vi "MB Director.vi"(4 "Timeout":u32=1000, 6 "MB Director":T1, 8 "error in (no error)":errorcluster, 11 "MB Port in":refnum<visa-resource-name>) -> (0 "error out":errorcluster, 3 "MB Port out":refnum<visa-resource-name>)   [LabVIEW 2019]
uses:
  MB Director.ctl
  MB cmd buffer.ctl
  MB Serial Master Query Write Multiple Registers (poly).vi
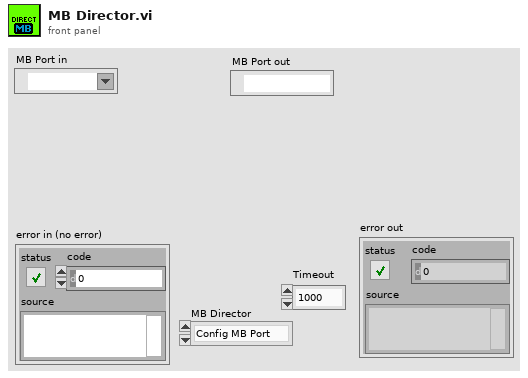
[diagram p1: front panel]
types:
  T1 = typedef "MB Director.ctl" = enum16{"Config MB Port", "Run MB", "Get MB Port", "Quit MB"}
  T2 = typedef "MB cmd buffer.ctl" = enum16{"ProCoDA", "MB", "MB Next Task", "ProCoDA read 1"}
  T3 = typedef "MB ID-Address.ctl" = cluster{"Device ID":u8, "Register":u16}
  T4 = typedef "MB status.ctl" = cluster{"ProCoDA Request":T5, "MB response":dbl[], "new cmd":bool, "error":errorcluster, "MB update(s)":dbl}
  T5 = typedef "ProCoDA MB Request.ctl" = cluster{"# registers":u8, "Data to write":u16[], "data interval (s)":dbl, "command":T6, "PC update (s)":dbl}
  T6 = typedef "Read Write.ctl" = enum16{"Read", "Write"}
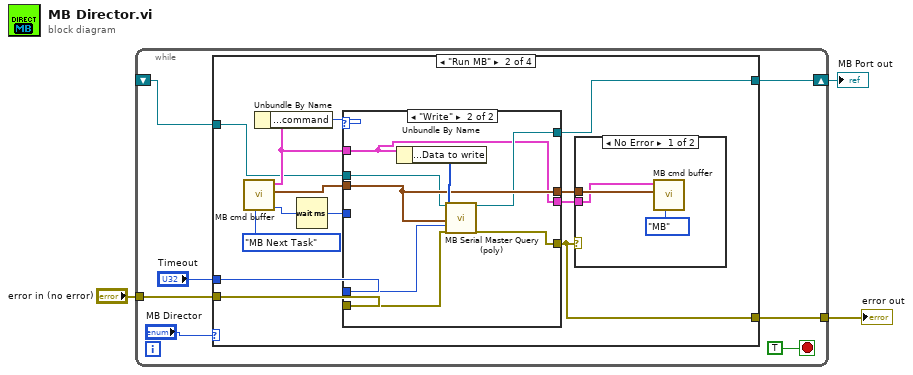
[diagram p0: block diagram]
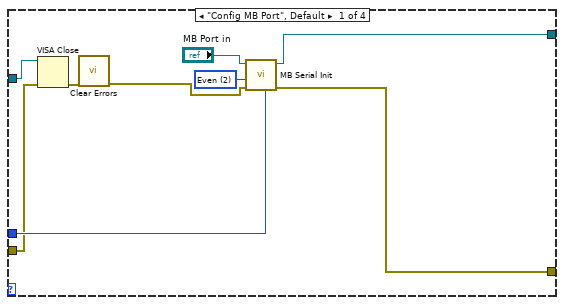
[diagram p2: hidden frame]
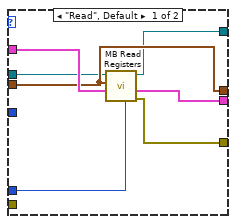
[diagram p4: hidden frame]
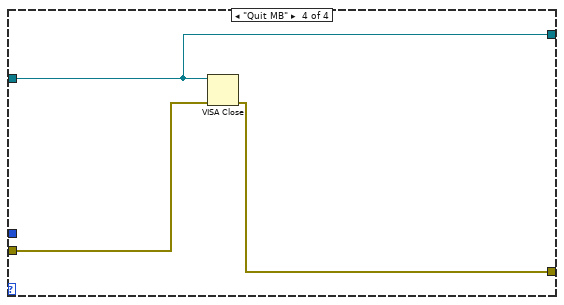
[diagram p6: hidden frame]
diagram:
  n1 = while {
    shift-right: [w5] -> w1
    shift-left: _ -> [w8]
    tunnel: "error in (no error)" -> [w7]
    tunnel: [w6] -> w2
    stop <- TRUE stop-if-true
    n2 = case shown="\"Run MB\"" "MB Director" {
      tunnel: w8 -> [w14 w23 w52 w53]
      tunnel: w7 -> [w13 w21 w51 w55]
      tunnel: [w16 w20 w51 w54] -> w6
      tunnel: [w19 w22 w52 w53] -> w5
      tunnel: "Timeout" -> [w17 w24 _ _]
      frame "Config MB Port", Default {
        w18 = u16 2 items=["None", "Odd", "Even", "Mark", "Space"] ("Parity")
        n3 = VISA Close(VISA resource name=w14, error in (no error)=w13) -> (error out=w12:errorcluster)
        n4 = call <vilib>:"Clear Errors.vi"("error in (no error)"=w12) -> ("error out"=w11:errorcluster)  [unwired: 5 in, 1 out]
        n5 = call "MB Serial Init.vi"("Timeout"=w17, "error in (no error)"=w11, "Parity"=w18, "VISA resource name"="MB Port in") -> ("error out"=w16:errorcluster, "VISA resource name out"=w19:refnum<visa-resource-name>)  [unwired: 6 in]
      }
      frame "Run MB" {
        n6 = call "MB cmd buffer.vi"("MB cmd buffer"=MB_cmd_buffer."MB Next Task") -> ("wait"=w28:i32, "MB ID-Address out"=w30:T3, "MB status out"=w29:T4)  [unwired: 6 in, 1 out]
        n7 = Unbundle By Name(w29) -> ("ProCoDA Request.command"=w31:T6)
        n8 = Wait (ms)(milliseconds to wait=w28) -> (millisecond timer value=w25:u32)
        n9 = case shown="\"Write\"" w31 {
          tunnel: w29 -> [w41 w43]
          tunnel: w30 -> [w39 w49]
          tunnel: [w39 w49] -> w27
          tunnel: [w38 w48] -> w20
          tunnel: w24 -> [w42 w47]
          tunnel: [w40 w43] -> w26
          tunnel: w25 -> [_ _]
          tunnel: w23 -> [w37 w46]
          tunnel: [w36 w45] -> w22
          tunnel: w21 -> [_ w44]
          frame "Read", Default {
            n10 = call "MB Read Registers.vi"("Timeout"=w42, "MB status in"=w41, "MB ID-Address"=w39, "VISA resource name"=w37) -> ("error out"=w38:errorcluster, "MB status out"=w40:T4, "VISA resource name out"=w36:refnum<visa-resource-name>)  [unwired: 3 in, 2 out]
          }
          frame "Write" {
            n11 = Unbundle By Name(w43) -> ("ProCoDA Request.Data to write"=w50:u16[])
            n12 = call-poly "MB Serial Master Query (poly).vi"("VISA resource name"=w46, "Registers"=w50, "MB ID-Address in"=w49, "Timeout"=w47, "error in"=w44) -> ("VISA resource name out"=w45:refnum<visa-resource-name>, "error out"=w48:errorcluster)  [unwired: 12 in, 1 out]
          }
        }
        n13 = case shown="No Error" w20 {
          tunnel: w27 -> [w34 _]
          tunnel: w26 -> [w33 _]
          frame No Error {
            n14 = call "MB cmd buffer.vi"("MB cmd buffer"=MB_cmd_buffer."MB", "MB ID-Address in"=w34, "MB status in"=w33) -> ()  [unwired: 4 in, 4 out]
          }
          frame Error {
          }
        }
      }
      frame "Get MB Port" {
      }
      frame "Quit MB" {
        n15 = VISA Close(VISA resource name=w53, error in (no error)=w55) -> (error out=w54:errorcluster)
      }
    }
  }
  "error out" <- w2
  "MB Port out" <- w1
